vi "CloseBkPrecisionInput.vi"(2 "error out 2":errorcluster, 3 "VISA resource name out 2":refnum<visa-resource-name>) -> (0 "error out":errorcluster, 1 "VISA resource name out":refnum<visa-resource-name>)   [LabVIEW 2010]
uses:
  <instrlib>/BK Precision 85XX Series/BK Precision 85XX Series.lvlib
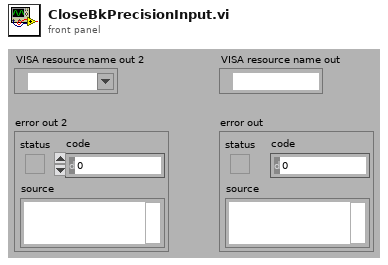
[diagram p1: front panel]
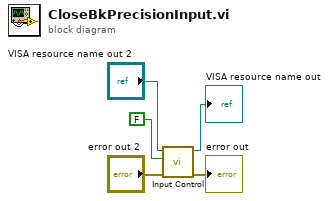
[diagram p0: block diagram]
diagram:
  n1 = call <instrlib>:"Input Control.vi"("error in (no error)"="error out 2", "Enable Input Terminals (F: Off)"=FALSE, "VISA resource name"="VISA resource name out 2") -> ("error out"=→"error out":errorcluster, "VISA resource name out"=→"VISA resource name out":refnum<visa-resource-name>)  [unwired: 7 in]
